vi "tearDown.vi"(8 "error in (no error)":errorcluster, 11 "reference in":refnum<class "NI-SWITCH Import Export Unit Tests.lvclass">) -> (0 "error out":errorcluster, 3 "reference out":refnum<class "NI-SWITCH Import Export Unit Tests.lvclass">)   [LabVIEW 2017, in "NI-SWITCH Import Export Unit Tests.lvclass"]
doc: "tearDown runs after the test method has completed. Use this method to clean up any operations or references that were opened by setUp or the test method. Unit tests should be independent of other unit tests so this VI should ensure that the next test can run in a 'clean' test environment."
uses:
  NI-SWITCH Import Export Unit Tests.lvclass
  NI-SWITCH Import Export Unit Tests.lvclass/NI-SWITCH Import Export Unit Tests.ctl
  NationalInstruments.VeriStand.SystemDefinitionAPI
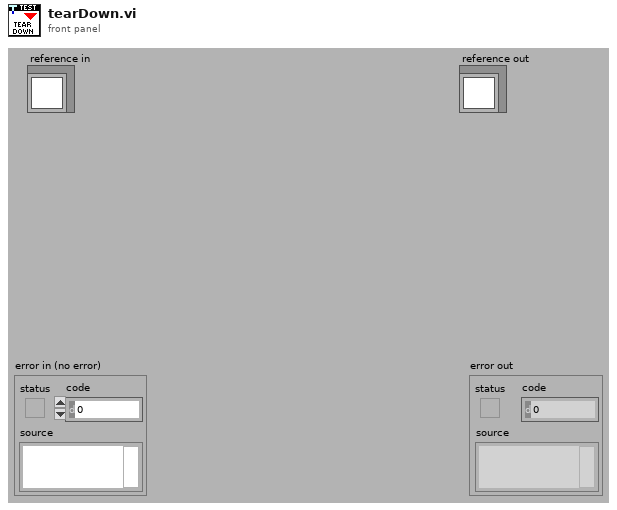
[diagram p1: front panel]
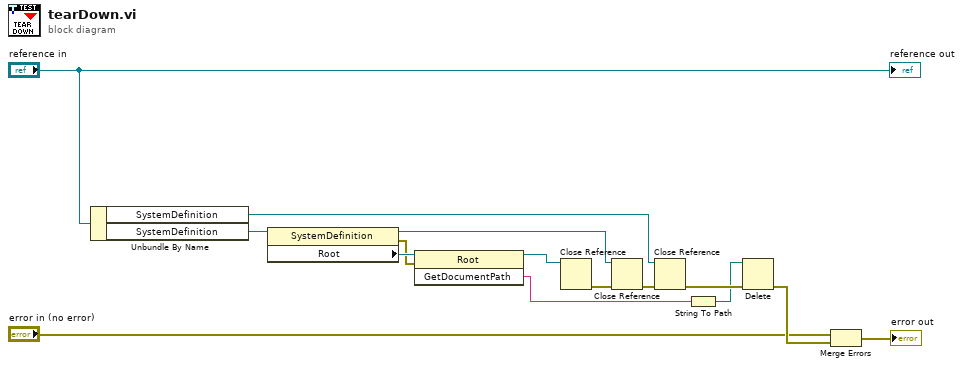
[diagram p0: block diagram]
diagram:
  n1 = Unbundle By Name("reference in") -> ("SystemDefinition"=w12:refnum<k24>, "SystemDefinition"=w10:refnum<k24>)
  n2 = property class="SystemDefinition"(reference=w10) -> (reference out=w11:refnum<k24>, error out=w8:errorcluster, "Root"=w9:refnum<k24>)  [unwired: 1 in]
  n3 = invoke class="Root" method="GetDocumentPath"(reference=w9, error in=w8) -> (reference out=w6:refnum<k24>, "GetDocumentPath"=w1:string)  [unwired: 1 in, 1 out]
  n4 = Close Reference(reference=w6) -> (error out=w7:errorcluster)  [unwired: 1 in]
  n5 = Close Reference(reference=w11, error in (no error)=w7) -> (error out=w14:errorcluster)
  n6 = Close Reference(reference=w12, error in (no error)=w14) -> (error out=w13:errorcluster)
  n7 = String To Path(string=w1) -> (path=w2:path)
  n8 = Delete(path (use dialog)=w2, error in=w13) -> (error out=w5:errorcluster)  [unwired: 3 in, 2 out]
  n9 = Merge Errors("error in (no error)", w5) -> (→"error out":errorcluster)
  "reference out" <- "reference in"
